vi "Teleop.vi"(10 "Wheels down":bool, 11 "shooter.lvclass":refnum<class "shooter.lvclass">) -> (3 "shooter.lvclass":refnum<class "shooter.lvclass">)   [LabVIEW 2015, in "shooter.lvclass"]
uses:
  shooter.lvclass
  Robot Global Data.vi
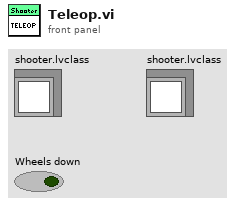
[diagram p1: front panel]
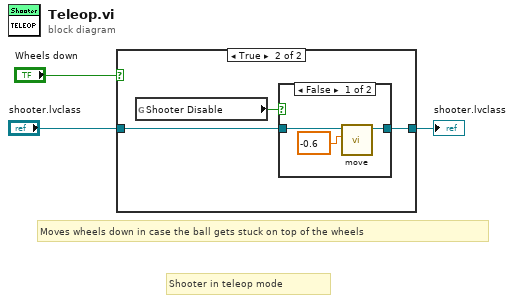
[diagram p0: block diagram]
diagram:
  # "Shooter in teleop mode"
  # "Moves wheels down in case the ball gets stuck on top of the wheels"
  n1 = case shown="True" "Wheels down" {
    tunnel: "shooter.lvclass" -> [w4 w6]
    tunnel: [w4 w5] -> w2
    frame False {
    }
    frame True {
      n2 = global read "Robot Global Data.vi" "Shooter Disable"() -> (w7:bool)
      n3 = case shown="False" w7 {
        tunnel: w6 -> [w9 w11]
        tunnel: [w8 w11] -> w5
        frame False {
          n4 = call "move.vi"("Speed"=-0.6 ("Right axis value"), "shooter.lvclass"=w9) -> ("shooter.lvclass"=w8:refnum<class "shooter.lvclass">)  [unwired: 9 in]
        }
        frame True {
        }
      }
    }
  }
  "shooter.lvclass" <- w2
